vi "Adv_GetControlCurrentCapabilities_alt.vi"(8 "error in (no error)":errorcluster, 9 "Setting":T1(ring), 10 "Control":refnum<vi>, 11 "LightField Automation in":refnum<class "LightField Automation.lvclass">) -> (0 "error out":errorcluster, 2 "Array":variant[](array[variant]), 3 "LightField Automation out":refnum<class "LightField Automation.lvclass">)   [LabVIEW 2013]
uses:
  C:/Program Files/Princeton Instruments/LightField/AddInViews/PrincetonInstruments.LightFieldViewV3.dll
  Program Files/Princeton Instruments/LightField/AddInViews/PrincetonInstruments.LightFieldViewV3.dll
  C:/Program Files/Princeton Instruments/LightField/PrincetonInstruments.LightFieldAddInSupportServices.dll
  Program Files/Princeton Instruments/LightField/PrincetonInstruments.LightFieldAddInSupportServices.dll
  LightField Automation.lvclass
panel:
  in  "UninitializedEnum":i32(ring) items=["UninitializedEnum", "LowNoise", "HighCapacity", "ElectronMultiplied", "HighSpeed"]
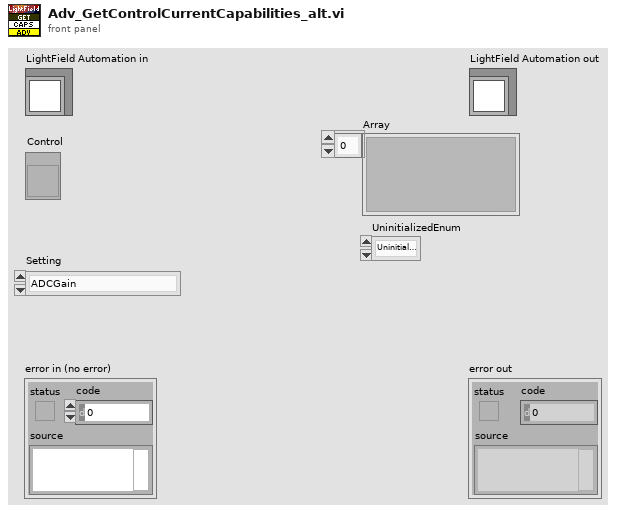
[diagram p1: front panel]
types:
  T1 = enum16{"ADCGain", "ADCQuality", "CalibrationLightSource", "CalibrationMode", "CcdCharacteristics", "CosmicRayCorrectionMethod", "DateFormat", "EMIccdGainControlMode", "FeatureProvider", "FileFormatLocation", "FrameCombinationMethod", "GateTracking", "GatingMode", "GatingSpeed", "IEMGainControlMode", "ImageOrientation", "IntensifierOptions", "IntensifierStatus", "ModulationTracking", "OpticalPortLocation", "OpticalPortShutterType", "OpticalPortType", "OutputSignal", "PhosphorType", "PhotocathodeSensitivity", "PhotonDetectionMode", "PixelDataFormat", "PixelFormat", "ReadoutControlMode", "ReadoutOrientation", "RegionsOfInterestSelection", "SensorTemperatureStatus", "SensorType", "ShutterAccessoryTimingMode", "ShutterTimingMode", "TimeFormat", "TimeStamps", "TriggerCoupling", "TriggerDetermination", "TriggerResponse", "TriggerSource", "TriggerTermination"}
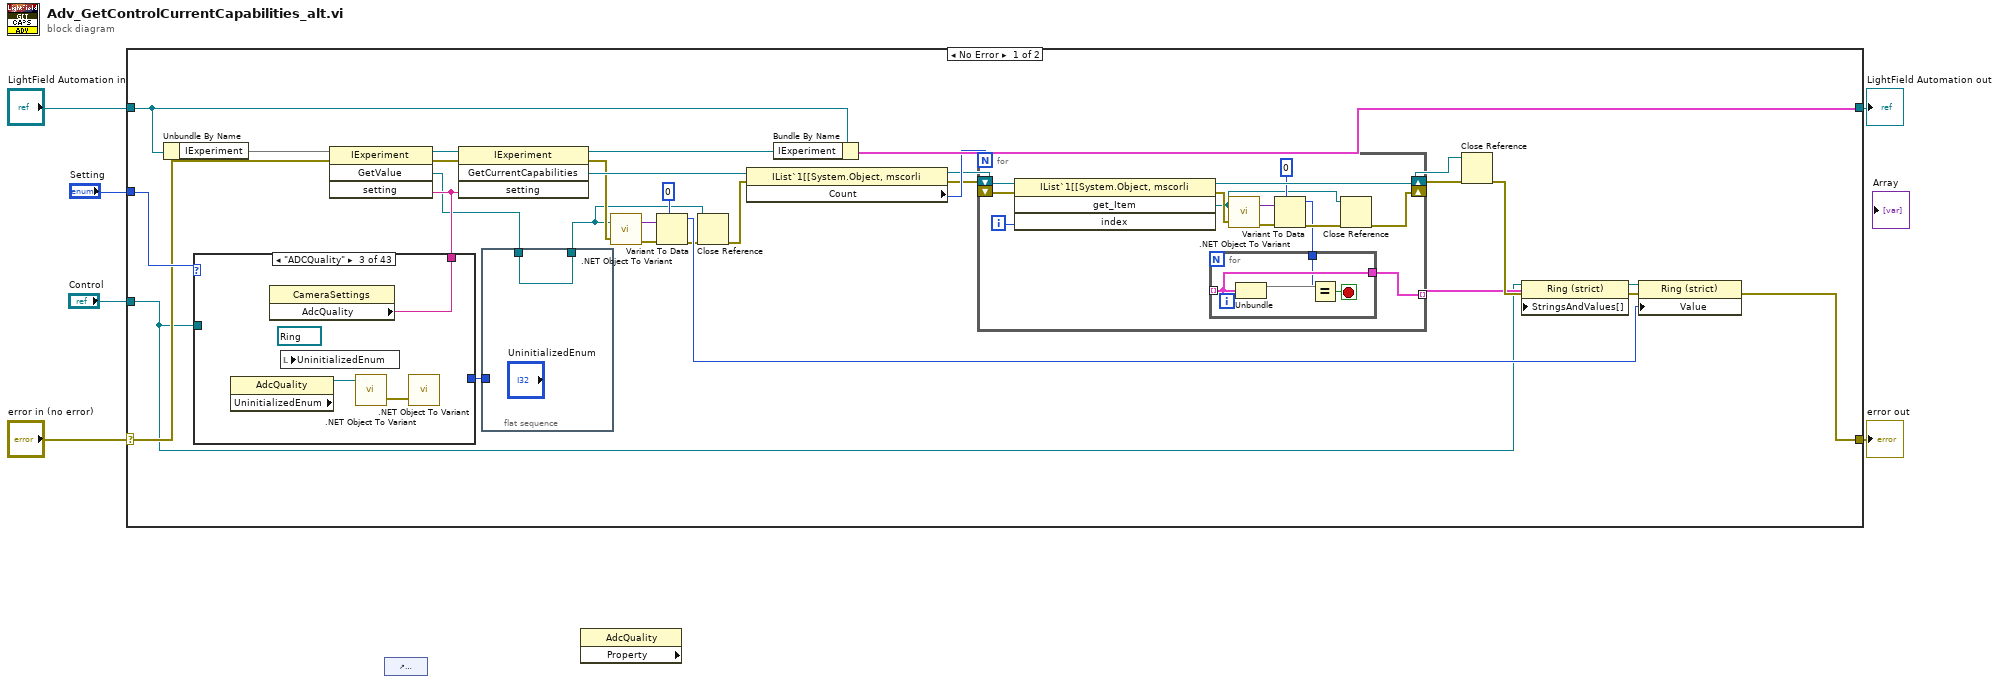
[diagram p0: block diagram]
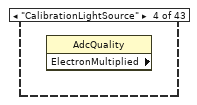
[diagram p4: hidden frame]
diagram:
  n1 = case shown="No Error" "error in (no error)" {
    selector: "error in (no error)" -> [w23 w61]
    tunnel: [w14 w61] -> w5
    tunnel: [w36 w60] -> w3
    tunnel: "LightField Automation in" -> [w37 w60]
    tunnel: "Control" -> [w7 _]
    tunnel: "Setting" -> [w28 _]
    frame No Error {
      n2 = Unbundle By Name(w37) -> ("IExperiment"=w26)
      n3 = case shown="\"ADCQuality\"" w28 {
        tunnel: [_ _ w41 _ _ _ _ _ _ _ _ _ _ _ _ _ _ _ _ _ _ _ _ _ _ _ _ _ _ _ _ _ _ _ _ _ _ _ _ _ _ _ _] -> w19
        tunnel: [_ _ _ _ _ _ _ _ _ _ _ _ _ _ _ _ _ _ _ _ _ _ _ _ _ _ _ _ _ _ _ _ _ _ _ _ _ _ _ _ _ _ _] -> w12
        tunnel: w7 -> [_ _ _ _ _ _ _ _ _ _ _ _ _ _ _ _ _ _ _ _ _ _ _ _ _ _ _ _ _ _ _ _ _ _ _ _ _ _ _ _ _ _ _]
        frame Default {
        }
        frame "ADCGain" {
        }
        frame "ADCQuality" {
          (unwired) refnum<vi> refnum ("Control")
          n4 = property class="AdcQuality" props=["UninitializedEnum"]() -> (reference out=w40:refnum<k24>)  [unwired: 2 in, 2 out]
          n5 = property class="CameraSettings"() -> ("AdcQuality"=w41:string)  [unwired: 2 in, 2 out]
          n6 = local read "UninitializedEnum"() -> ()  [unwired: 1 in]
          n7 = call <vilib>:".NET Object To Variant.vi"(".NET object"=w40) -> ("error out"=w39:errorcluster)  [unwired: 1 in, 1 out]
          n8 = call <vilib>:".NET Object To Variant.vi"("error in (no error)"=w39) -> ()  [unwired: 1 in, 2 out]
        }
        frame "CalibrationLightSource" {
          n9 = property class="AdcQuality" props=["ElectronMultiplied"]() -> ()  [unwired: 2 in, 3 out]
        }
        frame "CalibrationMode" {
        }
        frame "CcdCharacteristics" {
        }
        frame "CosmicRayCorrectionMethod" {
        }
        frame "DateFormat" {
        }
        frame "EMIccdGainControlMode" {
        }
        frame "FeatureProvider" {
        }
        frame "FileFormatLocation" {
        }
        frame "FrameCombinationMethod" {
        }
        frame "GateTracking" {
        }
        frame "GatingMode" {
        }
        frame "GatingSpeed" {
        }
        frame "IEMGainControlMode" {
        }
        frame "ImageOrientation" {
        }
        frame "IntensifierOptions" {
        }
        frame "IntensifierStatus" {
        }
        frame "ModulationTracking" {
        }
        frame "OpticalPortLocation" {
        }
        frame "OpticalPortShutterType" {
        }
        frame "OpticalPortType" {
        }
        frame "OutputSignal" {
        }
        frame "PhosphorType" {
        }
        frame "PhotocathodeSensitivity" {
        }
        frame "PhotonDetectionMode" {
        }
        frame "PixelDataFormat" {
        }
        frame "PixelFormat" {
        }
        frame "ReadoutControlMode" {
        }
        frame "ReadoutOrientation" {
        }
        frame "RegionsOfInterestSelection" {
        }
        frame "SensorTemperatureStatus" {
        }
        frame "SensorType" {
        }
        frame "ShutterAccessoryTimingMode" {
        }
        frame "ShutterTimingMode" {
        }
        frame "TimeFormat" {
        }
        frame "TimeStamps" {
        }
        frame "TriggerCoupling" {
        }
        frame "TriggerDetermination" {
        }
        frame "TriggerResponse" {
        }
        frame "TriggerSource" {
        }
        frame "TriggerTermination" {
        }
      }
      n10 = invoke class="IExperiment" method="GetValue"(reference=w26, error in=w23, "setting"=w19) -> (reference out=w25:refnum<k24>, error out=w24:errorcluster, "GetValue"=w8:refnum<k24>)  [unwired: 1 in, 1 out]
      n11 = invoke class="IExperiment" method="GetCurrentCapabilities"(reference=w25, error in=w24, "setting"=w19) -> (reference out=w27:refnum<k24>, error out=w11:errorcluster, "GetCurrentCapabilities"=w13:refnum<k24>)  [unwired: 1 in, 1 out]
      n12 = flat-sequence {
        tunnel: w12 -> [_]
        tunnel: [w38] -> w9
        tunnel: w8 -> [w38]
        frame #0 {
        }
      }
      n13 = call <vilib>:".NET Object To Variant.vi"("error in (no error)"=w11, ".NET object"=w9) -> ("error out"=w22:errorcluster, "variant"=w21:variant)
      n14 = Variant To Data(error in=w22, type=0, Variant=w21) -> (data=w16:i32, error out=w15:errorcluster)
      n15 = Close Reference(reference=w9, error in (no error)=w15) -> (error out=w10:errorcluster)
      n16 = property class="IList`1[[System.Object, mscorli"(reference=w13, error in=w10) -> (reference out=w34:refnum<k24>, error out=w33:errorcluster, "Count"=w35:i32)
      n17 = Bundle By Name(cluster=w37, "IExperiment"=w27) -> (w36:cluster{})
      n18 = for {
        N: w35 -> [_]
        shift-right: [w52] -> w31
        shift-left: w34 -> [w55]
        shift-right: [w46] -> w32
        shift-left: w33 -> [w54]
        tunnel: [w43] -> w29 mode=indexing
        i -> [w53]
        n19 = invoke class="IList`1[[System.Object, mscorli" method="get_Item"(reference=w55, error in=w54, "index"=w53) -> (reference out=w52:refnum<k24>, error out=w49:errorcluster, "get_Item"=w45:refnum<k24>)  [unwired: 1 in, 1 out]
        n20 = call <vilib>:".NET Object To Variant.vi"("error in (no error)"=w49, ".NET object"=w45) -> ("error out"=w51:errorcluster, "variant"=w50:variant)
        n21 = Variant To Data(error in=w51, type=0, Variant=w50) -> (data=w42:i32, error out=w47:errorcluster)
        n22 = for {
          tunnel: [w59] -> w44 mode=indexing
          tunnel: [w59] -> w43
          tunnel: w42 -> [w57]
          stop <- w56 stop-if-true
          n23 = Unbundle(w59) -> ("Value"=w58)  [unwired: 1 out]
          n24 = Equal?(x=w57, y=w58) -> (x = y?=w56:bool)
        }
        n25 = Close Reference(reference=w45, error in (no error)=w47) -> (error out=w46:errorcluster)
      }
      n26 = Close Reference(reference=w31, error in (no error)=w32) -> (error out=w30:errorcluster)
      n27 = property class="Ring (strict)"(reference=w7, error in=w30, "StringsAndValues[]"=w29) -> (reference out=w18:refnum<vi>, error out=w17:errorcluster)
      n28 = property class="Ring (strict)"(reference=w18, error in=w17, "Value"=w16) -> (error out=w14:errorcluster)  [unwired: 1 out]
    }
    frame Error {
    }
  }
  "error out" <- w5
  "LightField Automation out" <- w3
  n29 = control-ref of="UninitializedEnum"() -> ()  [unwired: 1 out]
  n30 = property class="AdcQuality" props=[]() -> ()  [unwired: 2 in, 3 out]
